vi "InterpAxis.vi"(0 "co-ord array":dbl[][](array[numeric]) format="%.5f", 1 "Invert Y ?":bool, 2 "z in":dbl[][](array[numeric]) format="%.4f", 3 "start value":dbl format="%.2e", 4 "Choose Pts?":bool, 5 "step size":dbl format="%.2e", 8 "PTs on Axis":u16[](array[numeric])) -> (6 "z interp":dbl[][](array[numeric]) format="%.5f")   [LabVIEW 2022 SP3]
panel:
  # "Start value is first value to start interpolating."
  # "step size increment to add to start value"
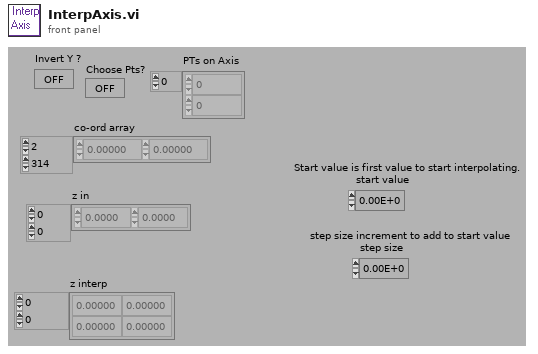
[diagram p1: front panel]
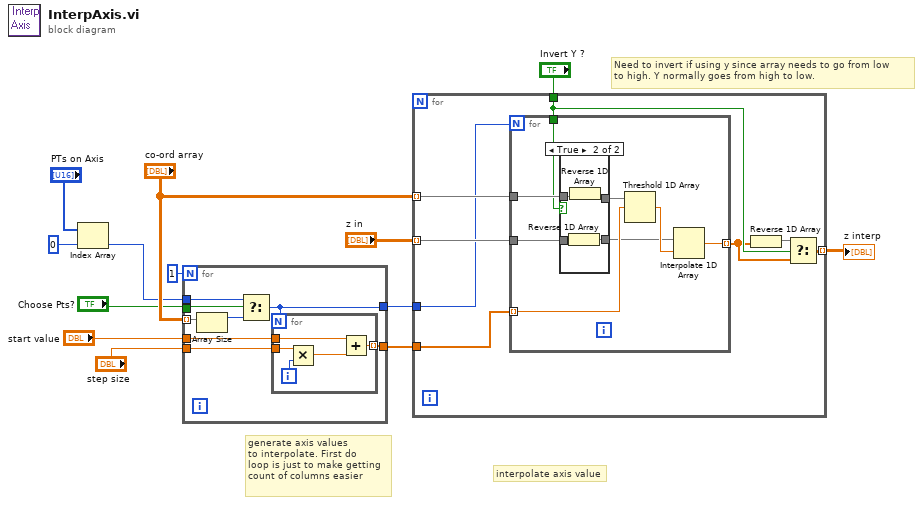
[diagram p0: block diagram]
diagram:
  # "Need to invert if using y since array needs to go from low\nto high. Y normally goes from high to low."
  # "interpolate axis value"
  # "generate axis values\nto interpolate. First do \nloop is just to make getting\ncount of columns easier"
  n1 = Index Array(array="PTs on Axis", index=0 ("Index")) -> (element=w3:u16)
  n2 = for {
    N: 1 -> [_]
    tunnel: "step size" -> [w21]
    tunnel: "start value" -> [w20]
    tunnel: [w19] -> w10
    tunnel: "co-ord array" -> [w18] mode=indexing
    tunnel: "Choose Pts?" -> [w17]
    tunnel: w3 -> [w15]
    tunnel: [w14] -> w1
    n3 = Array Size(array=w18) -> (size(s)=w16:i32)
    n4 = Select(t=w15, s=w17, f=w16) -> (s? t:f=w14:i32)
    n5 = for {
      N: w14 -> [_]
      tunnel: w21 -> [w25]
      tunnel: w20 -> [w23]
      tunnel: [w22] -> w19 mode=indexing
      i -> [w24]
      n6 = Multiply(x=w25, y=w24) -> (x*y=w26:dbl)
      n7 = Add(x=w23, y=w26) -> (x+y=w22:dbl)
    }
  }
  n8 = for {
    tunnel: "co-ord array" -> [w28] mode=indexing
    tunnel: "z in" -> [w34] mode=indexing
    tunnel: [w29] -> w8 mode=indexing
    tunnel: w10 -> [w33]
    tunnel: "Invert Y ?" -> [w31]
    tunnel: w1 -> [w27]
    n9 = for {
      N: w27 -> [_]
      tunnel: w28 -> [w37]
      tunnel: w34 -> [w39]
      tunnel: [w41] -> w30 mode=indexing
      tunnel: w33 -> [w40] mode=indexing
      tunnel: w31 -> [w35]
      n10 = case shown="True" w35 {
        tunnel: w39 -> [w43 w48]
        tunnel: [w43 w47] -> w38
        tunnel: w37 -> [w44 w46]
        tunnel: [w44 w45] -> w36
        frame False {
        }
        frame True {
          n11 = Reverse 1D Array(array=w48) -> (reversed array=w47:dbl[])
          n12 = Reverse 1D Array(array=w46) -> (reversed array=w45:dbl[])
        }
      }
      n13 = Threshold 1D Array(2:w40, 3:w36) -> (0:w42:dbl)  [unwired: 1 out]
      n14 = Interpolate 1D Array(1:w42, 2:w38) -> (0:w41:dbl)
    }
    n15 = Reverse 1D Array(array=w30) -> (reversed array=w32:dbl[])
    n16 = Select(t=w32, s=w31, f=w30) -> (s? t:f=w29:dbl[])
  }
  "z interp" <- w8
